vi "is a.vi"(8 "error in (no error)":errorcluster, 11 "CCD in":refnum<class "Motor.lvclass">) -> (0 "error out":errorcluster, 2 "is a":string, 3 "CCD out":refnum<class "Motor.lvclass">)   [LabVIEW 2016, in "Hardware.lvlib" / "Motor.lvlib" / "Motor.lvclass"]
uses:
  <userlib>/Common Components/Hardware/Motor/Motor/Motor.lvclass
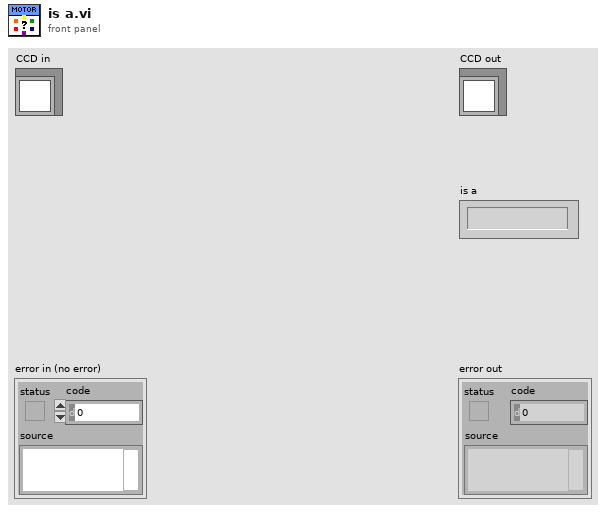
[diagram p1: front panel]
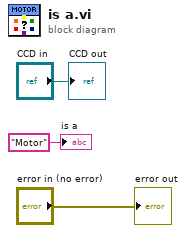
[diagram p0: block diagram]
diagram:
  "error out" <- "error in (no error)"
  "CCD out" <- "CCD in"
  "is a" <- "Motor" ("is a")
